vi "asset.create_begin.vi"(8 "error in":errorcluster, 10 "name":string, 11 "Client in":refnum<class "Client.lvclass">) -> (0 "error out":errorcluster, 2 "AssetCreateStaging":refnum<class "AssetCreateStaging.lvclass">, 3 "Client out":refnum<class "Client.lvclass">)   [LabVIEW 2020, in "Client.lvclass"]
doc: "Creates a new asset in Nominal with the given name and optional description, and returns a handle to it."
uses:
  Client.lvclass
  AssetCreateStaging/AssetCreateStaging.lvclass
  AssetCreateStaging/AssetCreateStaging.lvclass/AssetCreateStaging.ctl
  Client.lvclass/Client.ctl
  client.lvlib
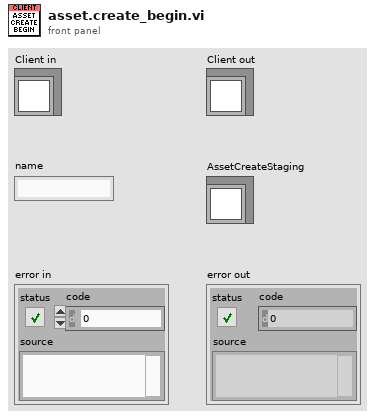
[diagram p1: front panel]
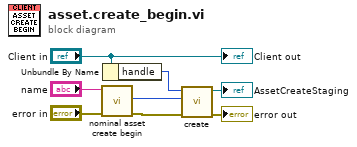
[diagram p0: block diagram]
diagram:
  n1 = call "nominal asset create begin.vi"("error in (no error)"="error in", "name"="name") -> ("error out"=w4:errorcluster, "out_staging out"=w6:i32)  [unwired: 7 in, 1 out]
  n2 = Unbundle By Name("Client in") -> ("handle"=w1:i32)
  n3 = call "create.vi"("error in (no error)"=w4, "handle"=w6, "client"=w1) -> ("error out"=→"error out":errorcluster, "AssetCreateStaging out"=→"AssetCreateStaging":refnum<class "AssetCreateStaging.lvclass">)  [unwired: 7 in]
  "Client out" <- "Client in"
